vi "Read 2D Array.vi"(8 "error in (no error)":errorcluster, 11 "Data2D in":refnum<class "Data2D.lvclass">) -> (0 "error out":errorcluster, 2 "2D Array":dbl[][](array[numeric]), 3 "Data2D out":refnum<class "Data2D.lvclass">)   [LabVIEW 2014, in "Data2D.lvclass"]
uses:
  Data2D.lvclass
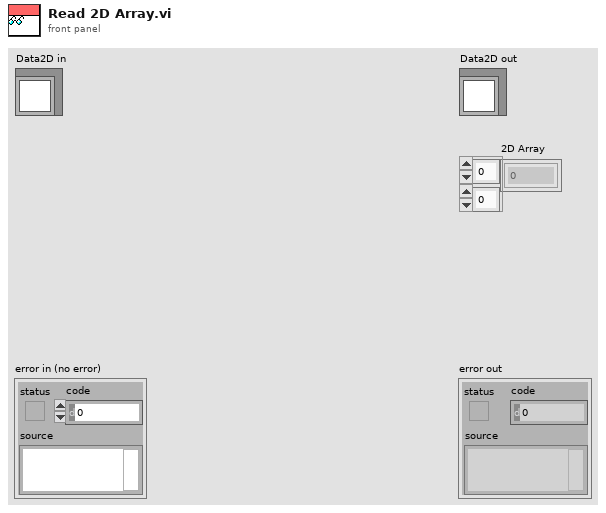
[diagram p1: front panel]
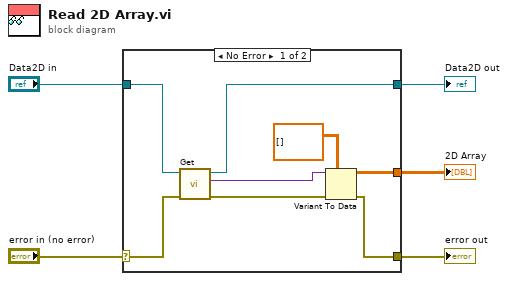
[diagram p0: block diagram]
diagram:
  n1 = case shown="No Error" "error in (no error)" {
    selector: "error in (no error)" -> [w9 w14]
    tunnel: [w7 w14] -> w4
    tunnel: [w6 w15] -> w2
    tunnel: "Data2D in" -> [w13 w15]
    tunnel: [w12 _] -> w1
    frame No Error {
      n2 = call-dynamic "Get.vi"("error in (no error)"=w9, "AbstractData in"=w13) -> ("error out"=w8:errorcluster, "Data"=w10:variant, "AbstractData out"=w6:refnum<class "Data2D.lvclass">)  [unwired: 7 in]
      n3 = Variant To Data(error in=w8, type=dbl[][] [] ("2D Array"), Variant=w10) -> (data=w12:dbl[][], error out=w7:errorcluster)
    }
    frame Error {
    }
  }
  "error out" <- w4
  "Data2D out" <- w2
  "2D Array" <- w1
